vi "TCP Msg Client.vi"() -> ()   [LabVIEW 2020]
uses:
  <vilib>/IlluminatedG/lv-stream-tcp/TCP Client/TCP Client.lvclass
  C:/Program Files (x86)/National Instruments/LabVIEW 2020/vi.lib/IlluminatedG/lv-stream/Endpoint/Endpoint.lvclass
  <vilib>/IlluminatedG/lv-stream/Endpoint/Endpoint.lvclass
  Manager/Manager.lvclass
panel:
  in  "Stop":bool
  out "error out":errorcluster
  out "Iteration":i32
  out "Slide":dbl(slide) scale=0.0..10.0
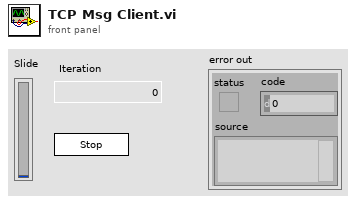
[diagram p1: front panel]
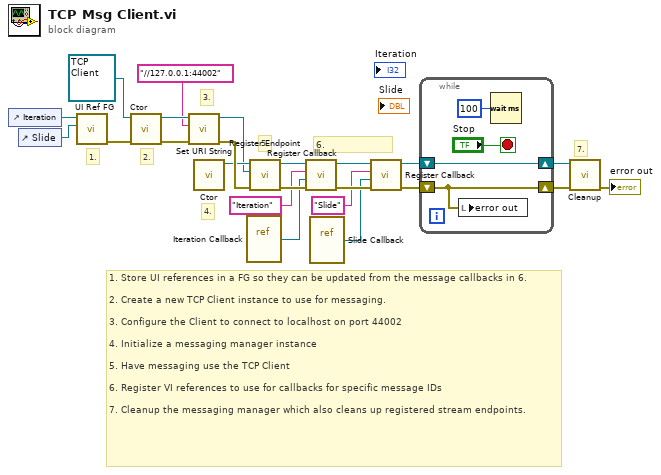
[diagram p0: block diagram]
diagram:
  # "1. Store UI references in a FG so they can be updated from the message callbacks in 6.\n\n2. Create a new TCP Client instance to use for messaging.\n\n3. Configure the Client to connect to localhost on port 44002\n\n4. Initialize a messaging manager instance\n\n5. Have messaging use the TCP Client\n\n6. Register VI references to use for callbacks for specific message IDs\n\n7. Cleanup the messaging manager which also cleans up registered stream endpoints."
  # "7."
  # "6."
  # "5."
  # "4."
  # "3."
  # "2."
  # "1."
  n1 = control-ref of="Iteration"() -> (w20:refnum<vi>)
  n2 = control-ref of="Slide"() -> (w19:refnum<vi>)
  n3 = call "UI Ref FG.vi"("Slide In"=w19, "Iteration In"=w20) -> ("error out"=w18:errorcluster)  [unwired: 7 in, 2 out]
  n4 = call-dynamic "Ctor.vi"("error in (no error)"=w18, "TCP Client in"=refnum<class "TCP Client.lvclass"> refnum) -> ("error out"=w15:errorcluster, "TCP Client out"=w16:refnum<class "TCP Client.lvclass">)  [unwired: 8 in]
  n5 = call <vilib>:"Set URI String.vi"("error in (no error)"=w15, "URI String"="//127.0.0.1:44002", "Endpoint in"=w16) -> ("error out"=w21:errorcluster, "Endpoint out"=w1:refnum<class "TCP Client.lvclass">)  [unwired: 7 in]
  n6 = call "Ctor.vi"() -> ("Manager out"=w13:refnum<class "Manager.lvclass">)  [unwired: 10 in, 1 out]
  n7 = vi-ref "Iteration Callback.vi"() -> (w10:refnum<vi>)
  n8 = call "Register Endpoint.vi"("error in (no error)"=w21, "Stream:Endpoint"=w1, "Manager in"=w13) -> ("error out"=w22:errorcluster, "Manager out"=w12:refnum<class "Manager.lvclass">)  [unwired: 7 in]
  n9 = call "Register Callback.vi"("error in (no error)"=w22, "Callback"=w10, "Message ID"="Iteration", "Manager in"=w12) -> ("error out"=w23:errorcluster, "Manager out"=w9:refnum<class "Manager.lvclass">)  [unwired: 6 in]
  n10 = vi-ref "Slide Callback.vi"() -> (w7:refnum<vi>)
  n11 = call "Register Callback.vi"("error in (no error)"=w23, "Callback"=w7, "Message ID"="Slide", "Manager in"=w9) -> ("error out"=w6:errorcluster, "Manager out"=w5:refnum<class "Manager.lvclass">)  [unwired: 6 in]
  n12 = while {
    shift-right: [w24] -> w4
    shift-left: w6 -> [w24]
    shift-right: [w27] -> w3
    shift-left: w5 -> [w27]
    stop <- "Stop" stop-if-true
    n13 = local write "error out"(w24) -> ()
    n14 = Wait (ms)(milliseconds to wait=u32 100) -> ()  [unwired: 1 out]
  }
  n15 = call "Cleanup.vi"("error in (no error)"=w4, "Manager in"=w3) -> ("error out"=→"error out":errorcluster)  [unwired: 9 in]
